vi "Find HW.vi"(8 "error in (no error)":errorcluster, 10 "HW Item":T1, 11 "Hardware Settings in":refnum<class "Hardware Settings.lvclass">) -> (0 "error out":errorcluster, 2 "Selected Hardware Out":refnum<class "Generic Hardware.lvclass">, 3 "Hardware Settings out":refnum<class "Hardware Settings.lvclass">)   [LabVIEW 2017, in "Hardware Settings.lvclass"]
uses:
  Hardware Settings.lvclass
  Type Defs/Hardware Types.ctl
  Hardware Types/Generic/Generic Hardware.lvclass
  Hardware Settings.lvclass/Hardware Settings.ctl
  Hardware Types/Generic/Generic Hardware.lvclass/Generic Hardware.ctl
  Hardware Types/Generic/Accessors/Read Description.vi
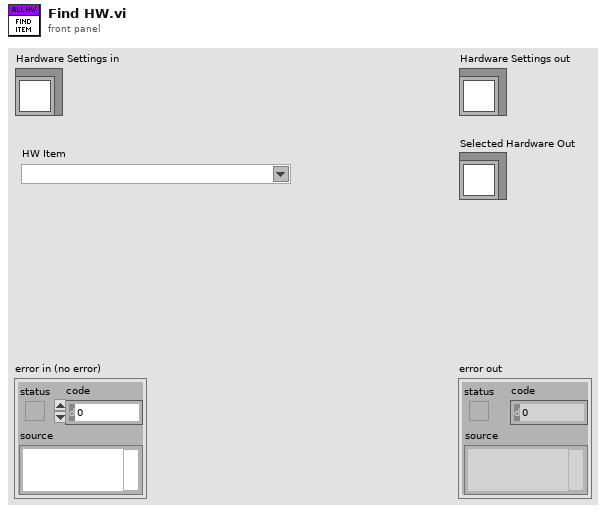
[diagram p1: front panel]
types:
  T1 = typedef "Hardware Settings.lvclass/Hardware Types.ctl" = string
  T2 = typedef "Hardware Types.ctl" = string
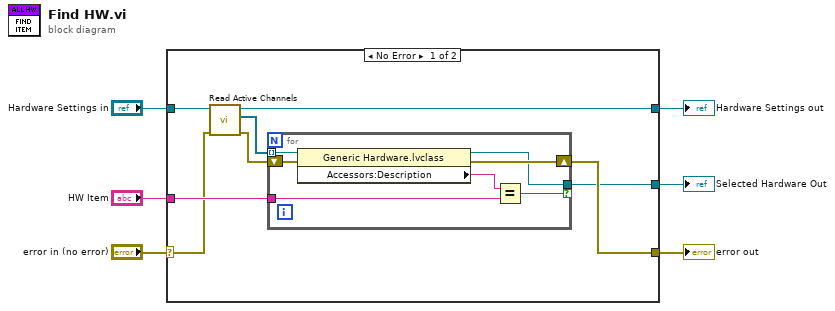
[diagram p0: block diagram]
diagram:
  n1 = case shown="No Error" "error in (no error)" {
    selector: "error in (no error)" -> [w10 w23]
    tunnel: [w8 w23] -> w5
    tunnel: [w13 w22] -> w3
    tunnel: "Hardware Settings in" -> [w14 w22]
    tunnel: "HW Item" -> [w11 _]
    tunnel: [w7 _] -> w1
    frame No Error {
      n2 = call "Read Active Channels.vi"("error in (no error)"=w10, "Hardware Settings in"=w14) -> ("error out"=w9:errorcluster, "Active Channels"=w12:refnum<class "Generic Hardware.lvclass">[], "Hardware Settings out"=w13:refnum<class "Hardware Settings.lvclass">)  [unwired: 7 in]
      n3 = for {
        tunnel: w12 -> [w21] mode=indexing
        tunnel: w11 -> [w19]
        shift-right: [w17] -> w8
        shift-left: w9 -> [w18]
        tunnel: [w15] -> w7 if=w16
        n4 = property class="Generic Hardware.lvclass"(reference=w21, error in=w18) -> (reference out=w15:refnum<class "Generic Hardware.lvclass">, error out=w17:errorcluster, "Accessors:Description"=w20:T2)
        n5 = Equal?(x=w20, y=w19) -> (x = y?=w16:bool)
      }
    }
    frame Error {
    }
  }
  "error out" <- w5
  "Hardware Settings out" <- w3
  "Selected Hardware Out" <- w1
